vi "Execute Device Command.vi"(0 "Session Handle in":T1, 5 "command":refnum<k21>, 11 "error in (no error)":errorcluster) -> (4 "Session Handle out":T1, 15 "error out":errorcluster)   [LabVIEW 2015]
uses:
  <vilib>/SLSC/SLSC.lvlib
  SLSC Session.lvclass
  Typedefs/Session Handle.ctl
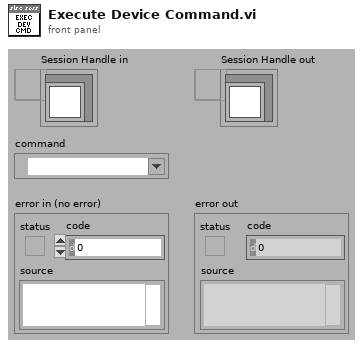
[diagram p1: front panel]
types:
  T1 = typedef "SLSC Switch.lvlib/SLSC Session.lvclass/Session Handle.ctl" = refnum<data-value>
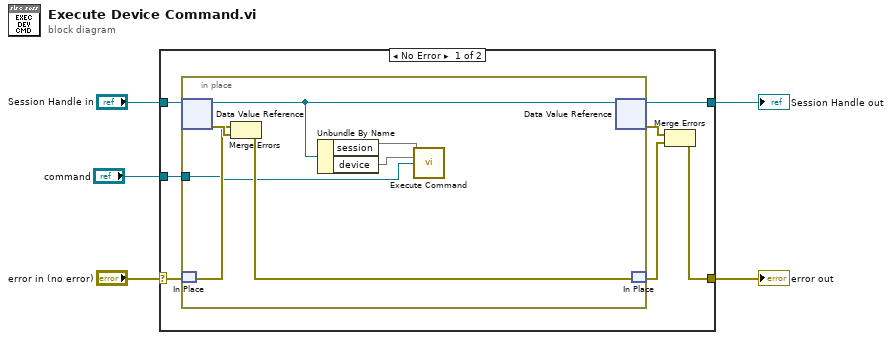
[diagram p0: block diagram]
diagram:
  n1 = case shown="No Error" "error in (no error)" {
    selector: "error in (no error)" -> [w7 w20]
    tunnel: "Session Handle in" -> [w12 w21]
    tunnel: [w11 w21] -> w4
    tunnel: [w8 w20] -> w3
    tunnel: "command" -> [w6 _]
    frame No Error {
      n2 = in-place {
        in-place-border: w6 -> [w13]
        n3 = in-place-dvr #1(w12) -> (w16:refnum<class "SLSC Session.lvclass">, w18:errorcluster)
        n4 = in-place-match #2(w7) -> (w17:errorcluster)
        n5 = Merge Errors(w17, w18) -> (w19:errorcluster)
        n6 = Unbundle By Name(w16) -> ("session"=w15, "device"=w14)
        n7 = call-poly <vilib>:"Execute Command.vi"("session in"=w15, "devices"=w14, "command"=w13) -> ()  [unwired: 11 in, 2 out]
        n8 = in-place-dvr #1(w16) -> (w11:T1, w9:errorcluster)
        n9 = in-place-match #2(w19) -> (w10:errorcluster)
      }
      n10 = Merge Errors(w9, w10) -> (w8:errorcluster)
    }
    frame Error {
    }
  }
  "Session Handle out" <- w4
  "error out" <- w3
